vi "Create global.vi"() -> ()   [LabVIEW 2019]
uses:
  Car Game/Supported.llb/Global-1.vi
  <vilib>/Utility/miscctls.llb/LVPointTypeDef.ctl
panel:
  in  "UP":bool
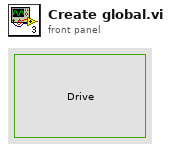
[diagram p1: front panel]
types:
  T1 = typedef "LVPointTypeDef.ctl" = cluster{"Horizontal":i16, "Vertical":i16}
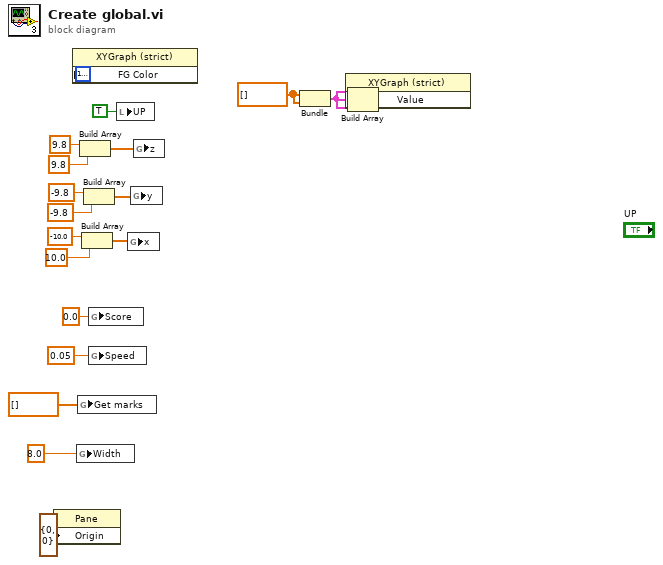
[diagram p0: block diagram]
diagram:
  w17 = dbl[] []
  n1 = property on="Property Node" class="Pane"("Origin"=T1 {"Horizontal"=0, "Vertical"=0}) -> ()  [unwired: 2 in, 2 out]
  n2 = property on="Property Node" class="XYGraph (strict)"("FG Color"=u32 16777216) -> ()  [unwired: 2 in, 2 out]
  n3 = global write "Global-1.vi" "Width"(8.0 ("opening width")) -> ()
  n4 = global write "Global-1.vi" "Get marks"(dbl[] []) -> ()
  n5 = Build Array(9.8 ("element"), 9.8 ("element")) -> (w7:dbl[])
  n6 = Build Array(-10.0 ("element"), 10.0 ("element")) -> (w9:dbl[])
  n7 = Build Array(-9.8 ("element"), -9.8 ("element")) -> (w8:dbl[])
  n8 = global write "Global-1.vi" "Score"(0.0 ("Score")) -> ()
  n9 = global write "Global-1.vi" "Speed"(0.05 ("Score")) -> ()
  n10 = local write "UP"(TRUE ("UP")) -> ()
  n11 = global write "Global-1.vi" "x"(w9) -> ()
  n12 = global write "Global-1.vi" "y"(w8) -> ()
  n13 = global write "Global-1.vi" "z"(w7) -> ()
  n14 = Bundle(w17, w17) -> (w18:cluster{dbl[], dbl[]})  [unwired: 1 in]
  n15 = Build Array(w18, w18, w18) -> (w19:cluster{dbl[], dbl[]}[])
  n16 = property on="Property Node" class="XYGraph (strict)"("Value"=w19) -> ()  [unwired: 2 in, 2 out]
